vi "Read Value.vi"(8 "Error In":errorcluster, 11 "Boolean In":refnum<class "Boolean.lvclass">) -> (0 "Error Out":errorcluster, 2 "Value":bool, 3 "Boolean Out":refnum<class "Boolean.lvclass">)   [LabVIEW 2018, in "Toolkit.lvlib" / "Data.lvlib" / "Boolean.lvclass"]
uses:
  Boolean.lvclass
  Boolean.lvclass/Boolean.ctl
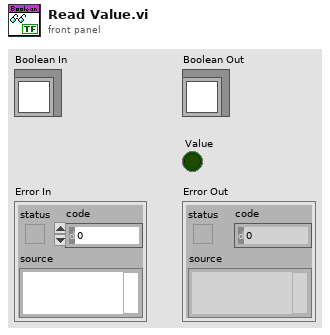
[diagram p1: front panel]
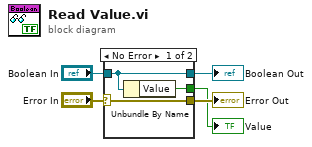
[diagram p0: block diagram]
diagram:
  n1 = case shown="No Error" "Error In" {
    selector: "Error In" -> [w8 w10]
    tunnel: [w8 w10] -> w4
    tunnel: "Boolean In" -> [w7 w9]
    tunnel: [w7 w9] -> w2
    tunnel: [w6 _] -> w1
    frame No Error {
      n2 = Unbundle By Name(w7) -> ("Value"=w6:bool)
    }
    frame Error {
    }
  }
  "Error Out" <- w4
  "Boolean Out" <- w2
  "Value" <- w1
